vi "Get Error Ring Info.vi"(8 "error in":errorcluster, 11 "Error VI Refnum":refnum<vi>) -> (0 "error out":errorcluster, 2 "Custom Description":string, 3 "code":i32)   [LabVIEW 2021, in "TAF Proj Document Type.lvlib" / "Project Parser.lvlib"]
uses:
  <vilib>/Wovalab/AntiDoc/Document Type/Add-ons/LabVIEW TAF Project/Project Parser/Project Parser.lvlib
  <vilib>/Utility/traverseref.llb/TRef TravTarget.ctl
  <vilib>/ErrorRing/Error Ring.ctl
  <vilib>/Utility/traverseref.llb/VI Scripting - Traverse.lvlib
  <vilib>/ErrorRing/Error Ring.xnode
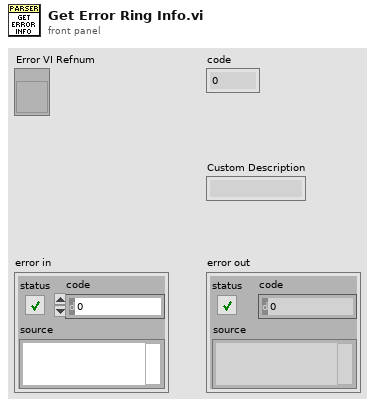
[diagram p1: front panel]
types:
  T1 = typedef "TRef TravTarget.ctl" = enum16{"FP", "BD", "Other"}
  T2 = typedef "Error Ring.xnode/Error Ring.ctl" = cluster{"Clipped Error Description":string, "Full Error Description":string, "code":i32, "Family":string, "Custom Description":string, "Is Error":bool, "Types":variant[], "Include Call Chain?":bool, "Error Text Visible":bool}
  T3 = cluster{"Library Version":cluster{"Major":u16, "Minor":u16, "Fix":u16, "Build":u16}, "State":variant}
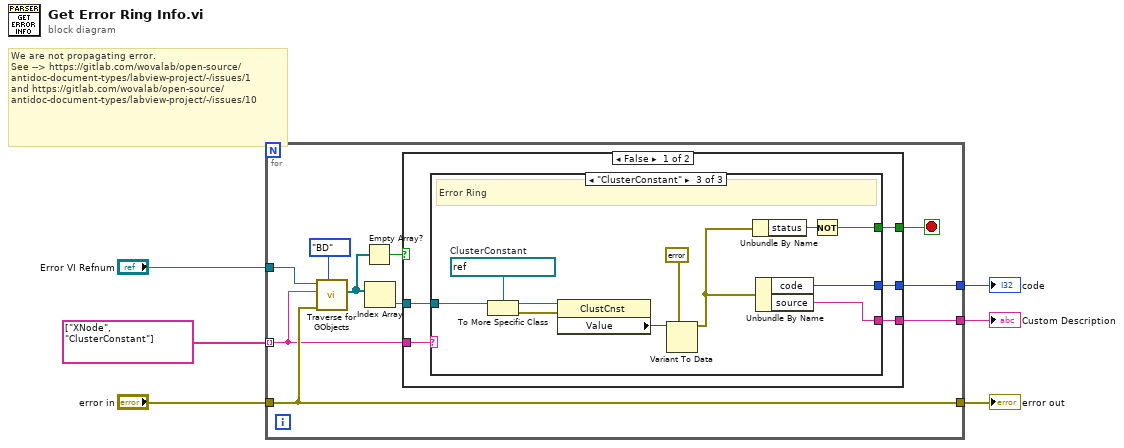
[diagram p0: block diagram]
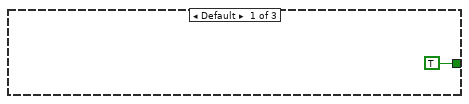
[diagram p2: hidden frame]
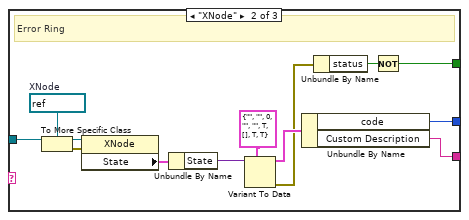
[diagram p3: hidden frame]
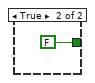
[diagram p4: hidden frame]
diagram:
  # "We are not propagating error.\nSee --> https://gitlab.com/wovalab/open-source/antidoc-document-types/labview-project/-/issues/1\nand https://gitlab.com/wovalab/open-source/antidoc-document-types/labview-project/-/issues/10"
  n1 = for {
    tunnel: [w15] -> w6
    tunnel: [w14] -> w5
    tunnel: "Error VI Refnum" -> [w13]
    tunnel: "error in" -> [w11]
    tunnel: [w11] -> w2
    tunnel: string[] ["XNode", "ClusterConstant"] -> [w8] mode=indexing
    stop <- w7 stop-if-true
    n2 = call <vilib>:"Traverse for GObjects.vi"("Traverse Target"=TRef_TravTarget."BD", "error in (no error)"=w11, "Class Name"=w8, "VI Refnum"=w13) -> ("References"=w10:refnum<vi>[])  [unwired: 4 in, 3 out]
    n3 = Empty Array?(array=w10) -> (empty?=w12:bool)
    n4 = Index Array(array=w10) -> (element=w9:refnum<vi>)  [unwired: 1 in]
    n5 = case shown="False" w12 {
      tunnel: [w21 _] -> w15
      tunnel: [w20 _] -> w14
      tunnel: w9 -> [w19 _]
      tunnel: w8 -> [w18 _]
      tunnel: [w17 FALSE] -> w7
      frame False {
        n6 = case shown="\"ClusterConstant\"" w18 {
          tunnel: [_ w28 w43] -> w21
          tunnel: [_ w27 w42] -> w20
          tunnel: w19 -> [_ w26 w41]
          tunnel: [TRUE w23 w37] -> w17
          frame Default {
          }
          frame "XNode" {
            w34 = refnum<vi> refnum  # XNode
            # "Error Ring"
            n7 = To More Specific Class(target class=w34, reference=w26) -> (specific class reference=w32:refnum<vi>, error out=w35:errorcluster)  [unwired: 1 in]
            n8 = property class="XNode"(reference=w32, error in=w35) -> ("State"=w31:T3)  [unwired: 2 out]
            n9 = Unbundle By Name(w31) -> ("State"=w33:variant)
            n10 = Variant To Data(type=T2 {"Clipped Error Description"="", "Full Error Description"="", "code"=0, "Family"="", "Custom Description"="", "Is Error"=TRUE, "Types"=[], "Include Call Chain?"=TRUE, "Error Text Visible"=TRUE} ("State"), Variant=w33) -> (data=w29:T2, error out=w25:errorcluster)  [unwired: 1 in]
            n11 = Unbundle By Name(w29) -> ("code"=w28:i32, "Custom Description"=w27:string)
            n12 = Unbundle By Name(w25) -> ("status"=w24:bool)
            n13 = Not(x=w24) -> (.not. x?=w23:bool)
          }
          frame "ClusterConstant" {
            w45 = refnum<vi> refnum  # ClusterConstant
            # "Error Ring"
            n14 = To More Specific Class(target class=w45, reference=w41) -> (specific class reference=w44:refnum<vi>, error out=w46:errorcluster)  [unwired: 1 in]
            n15 = property class="ClustCnst"(reference=w44, error in=w46) -> ("Value"=w40:variant)  [unwired: 2 out]
            n16 = Variant To Data(type=errorcluster {"status"=FALSE, "code"=0, "source"=""} ("error in (no error)"), Variant=w40) -> (data=w36:errorcluster)  [unwired: 1 in, 1 out]
            n17 = Unbundle By Name(w36) -> ("status"=w38:bool)
            n18 = Unbundle By Name(w36) -> ("code"=w43:i32, "source"=w42:string)
            n19 = Not(x=w38) -> (.not. x?=w37:bool)
          }
        }
      }
      frame True {
      }
    }
  }
  "code" <- w6
  "Custom Description" <- w5
  "error out" <- w2
